vi "UserView_WashDisplay_Console.vi"(8 "error in":errorcluster) -> (0 "error out":errorcluster)   [LabVIEW 2019]
uses:
  #typedef_Queue_enum.ctl
  #typedef_Data_Cluster.ctl
  #typedef_EntryConsole_Action_enum.ctl
  #typedef_WashDisplay_Action_enum.ctl
  #typedef_Controller_Action_enum.ctl
  #typedef_VehiclePosition_Action_enum.ctl
panel:
  out "Vehicle Out of Position":bool
  out "Time Remaining":string
  out "Wash Entry":string
  out "Air Dry":bool
  out "Under Body Wash":bool
  out "Bug Remover":bool
  out "Pre-Soak":bool
  out "High Pressure Wash (default)":bool
  out "Low Pressure Wax":bool
  out "Spot Free Rinse":bool
  out "Tire Shine Foam":bool
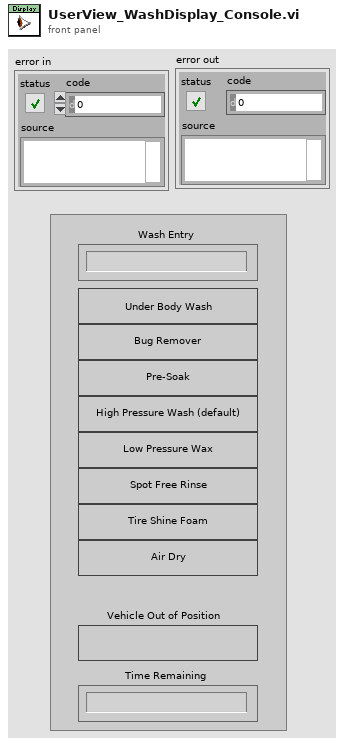
[diagram p1: front panel]
types:
  T1 = typedef "#typedef_Queue_enum.ctl" = enum16{"ERROR_default", "Obtain", "Enqueue", "GetStatus", "Flush", "Release"}
  T2 = typedef "#typedef_Data_Cluster.ctl" = cluster{"Dummy":dbl, "EntryConsole_Action":T3, "WashDisplay_Action":T4, "Controller_Action":T5, "VehiclePosition_Action":T6, "Wash Diplay Closed?":bool, "User Entry Closed?":bool, "Vehicle Pos Closed? ":bool}
  T3 = typedef "#typedef_EntryConsole_Action_enum.ctl" = enum16{"Init", "ERROR_DEFAULT", "Idle", "Specific", "Close", "Error_Handler", "Exit"}
  T4 = typedef "#typedef_WashDisplay_Action_enum.ctl" = enum16{"Init", "ERROR_DEFAULT", "Idle", "Specific", "Close", "Error_Handler", "Exit"}
  T5 = typedef "#typedef_Controller_Action_enum.ctl" = enum16{"Init", "ERROR_DEFAULT", "Idle", "Read database", "Close", "Error_Handler", "Exit"}
  T6 = typedef "#typedef_VehiclePosition_Action_enum.ctl" = enum16{"Init", "ERROR_DEFAULT", "Idle", "Specific", "Close", "Error_Handler", "Exit"}
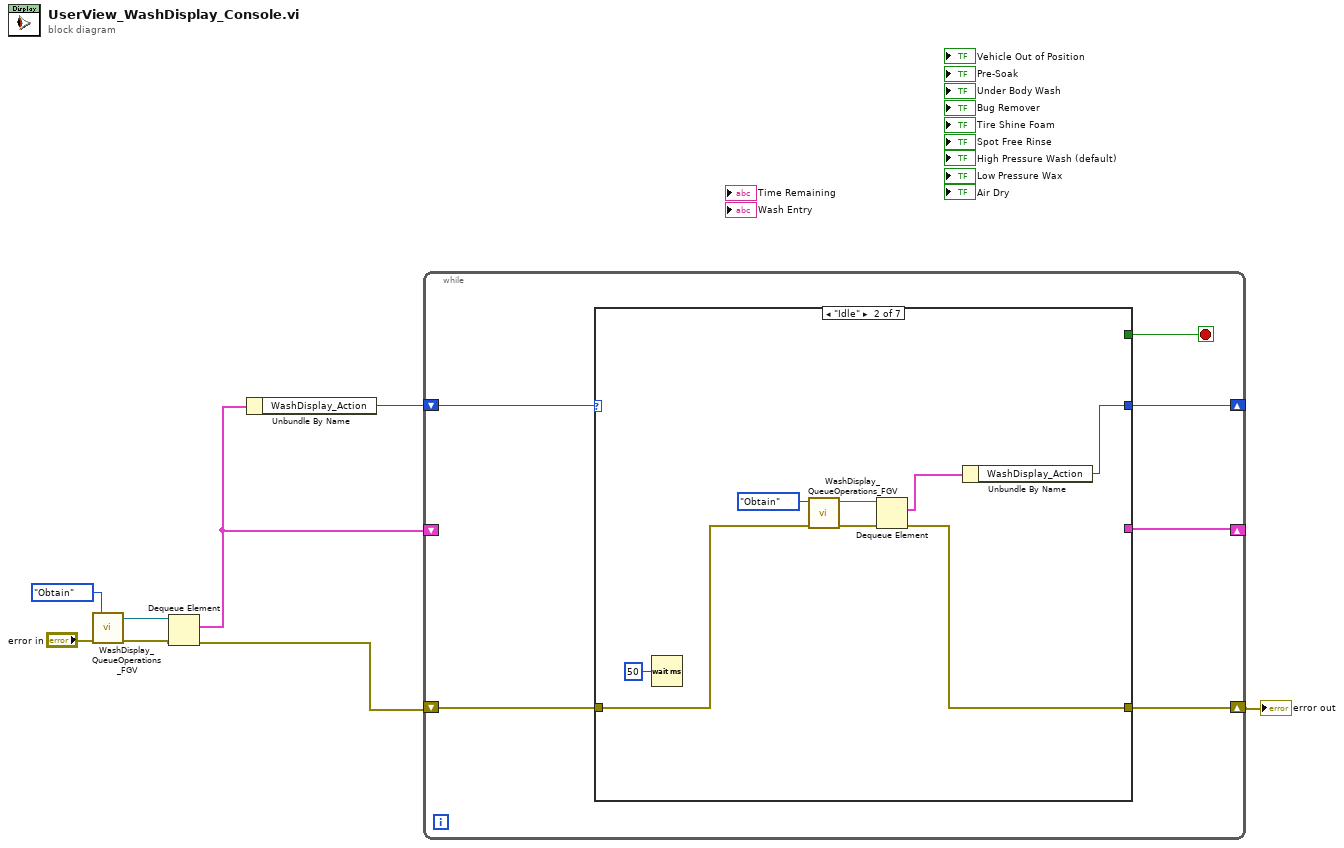
[diagram p0: block diagram]
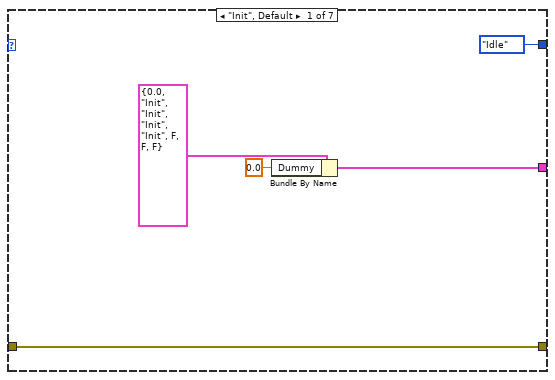
[diagram p2: hidden frame]
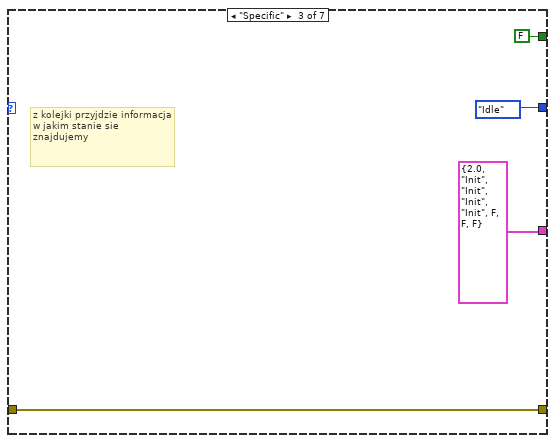
[diagram p3: hidden frame]
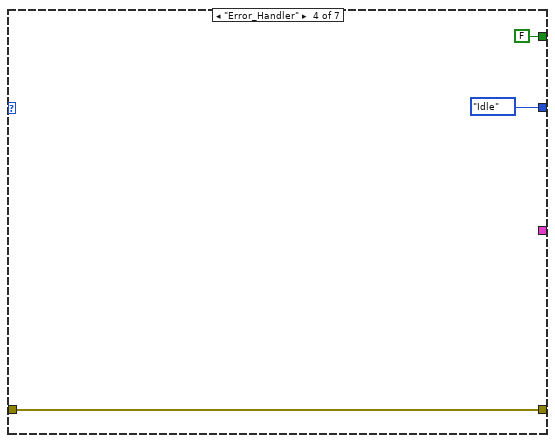
[diagram p4: hidden frame]
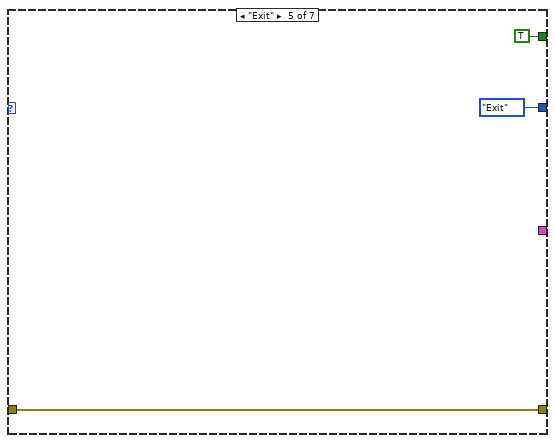
[diagram p5: hidden frame]
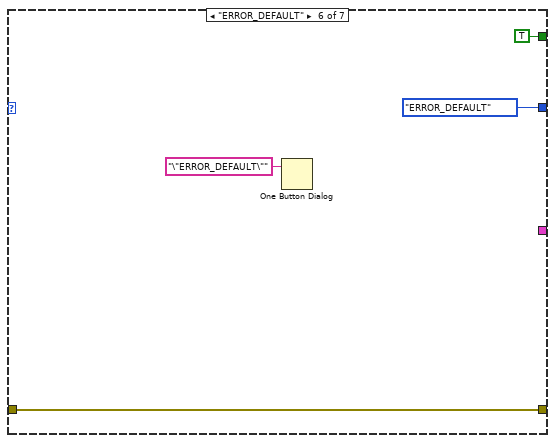
[diagram p6: hidden frame]
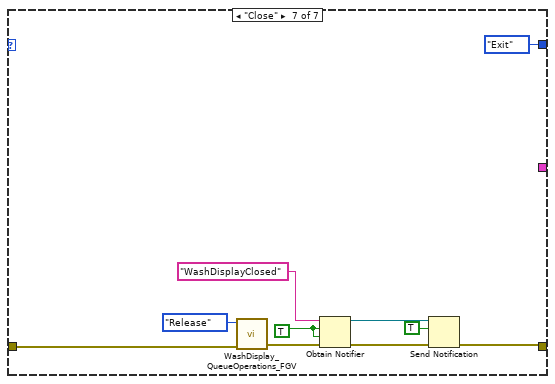
[diagram p7: hidden frame]
diagram:
  n1 = call "WashDisplay_QueueOperations_FGV.vi"("error in"="error in", "Action"=#typedef_Queue_enum."Obtain") -> ("error out"=w6:errorcluster, "queue ref"=w7:refnum<queue>)  [unwired: 6 in, 2 out]
  n2 = Dequeue Element(queue=w7, error in (no error)=w6) -> (element=w3:T2, error out=w4:errorcluster)  [unwired: 1 in, 2 out]
  n3 = Unbundle By Name(w3) -> ("WashDisplay_Action"=w2:T4)
  n4 = while {
    shift-right: [w13] -> _
    shift-left: w2 -> [w14]
    shift-right: [w11] -> _
    shift-left: w3 -> [_]
    shift-right: [w9] -> w1
    shift-left: w4 -> [w10]
    stop <- w12 stop-if-true
    n5 = case shown="\"Idle\"" w14 {
      tunnel: [#typedef_WashDisplay_Action_enum."Idle" ("WashDisplay_Action") w23 #typedef_WashDisplay_Action_enum."Idle" ("WashDisplay_Action") #typedef_WashDisplay_Action_enum."Idle" ("WashDisplay_Action") #typedef_WashDisplay_Action_enum."Exit" ("WashDisplay_Action") #typedef_WashDisplay_Action_enum."ERROR_DEFAULT" ("WashDisplay_Action") #typedef_WashDisplay_Action_enum."Exit" ("WashDisplay_Action")] -> w13
      tunnel: [_ _ FALSE FALSE TRUE TRUE _] -> w12
      tunnel: [w18 _ T2 {"Dummy"=2.0, "EntryConsole_Action"=enum."Init", "WashDisplay_Action"=enum."Init", "Controller_Action"=enum."Init", "VehiclePosition_Action"=enum."Init", "Wash Diplay Closed?"=FALSE, "User Entry Closed?"=FALSE, "Vehicle Pos Closed? "=FALSE} _ _ _ _] -> w11
      tunnel: w10 -> [w16 w26 w30 w33 w36 w39 w50]
      tunnel: [w16 w22 w30 w33 w36 w39 w44] -> w9
      frame "Init", Default {
        n6 = Bundle By Name(cluster=T2 {"Dummy"=0.0, "EntryConsole_Action"=enum."Init", "WashDisplay_Action"=enum."Init", "Controller_Action"=enum."Init", "VehiclePosition_Action"=enum."Init", "Wash Diplay Closed?"=FALSE, "User Entry Closed?"=FALSE, "Vehicle Pos Closed? "=FALSE}, "Dummy"=0.0) -> (w18:T2)
      }
      frame "Idle" {
        n7 = Wait (ms)(milliseconds to wait=u32 50) -> ()  [unwired: 1 out]
        n8 = call "WashDisplay_QueueOperations_FGV.vi"("error in"=w26, "Action"=#typedef_Queue_enum."Obtain") -> ("error out"=w25:errorcluster, "queue ref"=w21:refnum<queue>)  [unwired: 6 in, 2 out]
        n9 = Dequeue Element(queue=w21, error in (no error)=w25) -> (element=w20:T2, error out=w22:errorcluster)  [unwired: 1 in, 2 out]
        n10 = Unbundle By Name(w20) -> ("WashDisplay_Action"=w23:T4)
      }
      frame "Specific" {
        # "z kolejki przyjdzie informacja w jakim stanie sie znajdujemy"
      }
      frame "Error_Handler" {
      }
      frame "Exit" {
      }
      frame "ERROR_DEFAULT" {
        n11 = One Button Dialog(message="\"ERROR_DEFAULT\"") -> ()  [unwired: 1 in, 1 out]
      }
      frame "Close" {
        w46 = TRUE
        n12 = call "WashDisplay_QueueOperations_FGV.vi"("error in"=w50, "Action"=#typedef_Queue_enum."Release") -> ("error out"=w48:errorcluster)  [unwired: 6 in, 3 out]
        n13 = Obtain Notifier(name (unnamed)="WashDisplayClosed", notification data type=w46, create if not found? (T)=w46, error in (no error)=w48) -> (notifier out=w43:refnum<notifier>, error out=w45:errorcluster)  [unwired: 1 out]
        n14 = Send Notification(notification=TRUE, notifier=w43, error in (no error)=w45) -> (error out=w44:errorcluster)  [unwired: 1 out]
      }
    }
  }
  "error out" <- w1
